vi "Test Namer With Folder Creates Folder.vi"(11 "Test Case In":refnum<class "Namer Tests.lvclass">) -> (0 "error out":errorcluster, 3 "Test Case Out":refnum<class "Namer Tests.lvclass">)   [LabVIEW 2020, in "Namer Tests.lvclass"]
uses:
  Namer Tests.lvclass
  C:/Program Files/National Instruments/LabVIEW 2026/vi.lib/Astemes/LUnit/Test Case.lvclass
  Source/Approval Tests/Namer with Folder/Namer with Folder.lvclass
  Source/Approval Tests/Naming Data/Naming Data.lvclass
  Source/Approval Tests/Naming Data/Naming Data.lvclass/Naming Data.ctl
  <vilib>/Astemes/LUnit/Test Case.lvclass/Test Case.ctl
  01b65d38-618d-4a61-b092-aeaffa944d44.vi
  62f3f5be-2136-4147-be65-cbbff562f146.vi
  Source/Approval Tests/Naming Data/Write Test VI Name.vi
  <vilib>/Astemes/LUnit/Core/LUnit Test Case/Private/Append Pass Result.vi
  <vilib>/Astemes/LUnit/Core/LUnit Test Case/Private/Append Fail Result.vi
  01b65d38-618d-4a61-b092-aeaffa944d44.vi/9c5d11cd-9439-4240-a1ee-d9baace9c924.vi
  62f3f5be-2136-4147-be65-cbbff562f146.vi/9c5d11cd-9439-4240-a1ee-d9baace9c924.vi
  <vilib>/Astemes/LUnit/Core/LUnit Test Case/Private/Run In UI.vi
  <vilib>/Astemes/LUnit/Test Case.lvclass
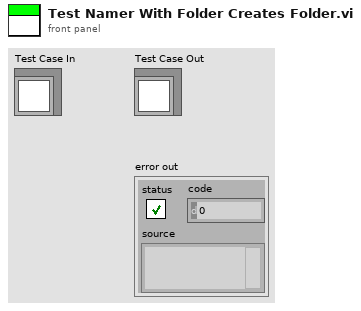
[diagram p1: front panel]
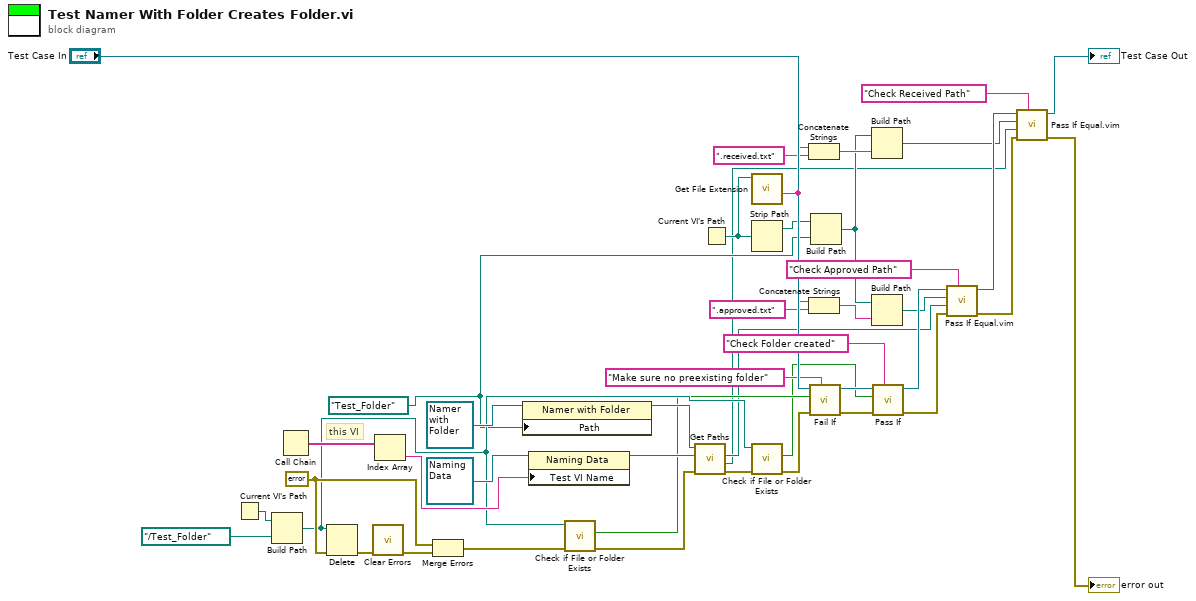
[diagram p0: block diagram]
diagram:
  w14 = path "Test_Folder" ("Path")
  w34 = errorcluster {"status"=FALSE, "code"=0, "source"=""} ("error in (no error)")
  # "this VI"
  n1 = Current VI's Path() -> (path=w35:path)
  n2 = Build Path(base path=w35, name or relative path=path "../Test_Folder") -> (appended path=w28:path)
  n3 = Call Chain() -> (call chain=w40:string[])
  n4 = Delete(path (use dialog)=w28, error in=w34) -> (error out=w33:errorcluster)  [unwired: 3 in, 2 out]
  n5 = call <vilib>:"Clear Errors.vi"("error in (no error)"=w33) -> ("error out"=w32:errorcluster)  [unwired: 5 in, 1 out]
  n6 = Index Array(array=w40) -> (element=w39:string)  [unwired: 1 in]
  n7 = Merge Errors(w34, w32) -> (w30:errorcluster)
  n8 = property class="Namer with Folder"(reference=refnum<class "Namer with Folder.lvclass"> refnum ("Approval Tests:Namer with Folder.lvclass"), "Path"=w14) -> (reference out=w37:refnum<class "Namer with Folder.lvclass">)  [unwired: 1 in, 1 out]
  n9 = property on="Property Node" class="Naming Data"(reference=refnum<class "Naming Data.lvclass"> refnum ("Naming Data"), "Test VI Name"=w39) -> (reference out=w38:refnum<class "Naming Data.lvclass">)  [unwired: 1 in, 1 out]
  n10 = call <vilib>:"Check if File or Folder Exists.vi"("error in (no error)"=w30, "path"=w28) -> ("error out"=w29:errorcluster, "file or folder exists?"=w27:bool)  [unwired: 7 in, 1 out]
  n11 = call-dynamic "Get Paths.vi"("error in"=w29, "Naming Data"=w38, "Namer with Folder in"=w37) -> ("error out"=w31:errorcluster, "Received Path"=w5:path, "Approved Path"=w6:path)  [unwired: 5 in, 1 out]
  n12 = Current VI's Path() -> (path=w22:path)
  n13 = call <vilib>:"Get File Extension.vi"("file"=w22) -> ("filename without extension"=w21:string)  [unwired: 6 in, 4 out]
  n14 = Strip Path(path=w22) -> (stripped path=w15:path)  [unwired: 1 out]
  n15 = call <vilib>:"Check if File or Folder Exists.vi"("error in (no error)"=w31, "path"=w28) -> ("error out"=w13:errorcluster, "file or folder exists?"=w23:bool)  [unwired: 7 in, 1 out]
  n16 = Concatenate Strings(w21, ".received.txt" ("string")) -> (w18:string)
  n17 = Concatenate Strings(w21, ".approved.txt" ("string")) -> (w17:string)
  n18 = call <vilib>:"Fail If.vi"("Description"="Make sure no preexisting folder" ("Label"), "error in (no error)"=w13, "Fail?"=w27, "LUnit Test Case In"="Test Case In") -> ("error out"=w43:errorcluster, "LUnit Test Case Out"=w25:refnum<class "Namer Tests.lvclass">)  [unwired: 6 in]
  n19 = Build Path(base path=w15, name or relative path=w14) -> (appended path=w16:path)
  n20 = Build Path(base path=w16, name or relative path=w18) -> (appended path=w4:path)
  n21 = Build Path(base path=w16, name or relative path=w17) -> (appended path=w3:path)
  n22 = call <vilib>:"Pass If.vi"("Description"="Check Folder created" ("Label (VI Title)"), "error in (no error)"=w43, "Pass?"=w23, "LUnit Test Case In"=w25) -> ("error out"=w8:errorcluster, "LUnit Test Case Out"=w12:refnum<class "Namer Tests.lvclass">)  [unwired: 6 in]
  n23 = call "Pass If Equal.vim"("Description"="Check Approved Path", "error in (no error)"=w8, "Actual"=w6, "Expected"=w3, "LUnit Test Case In"=w12) -> ("error out"=w7:errorcluster, "LUnit Test Case Out"=w10:refnum<class "Namer Tests.lvclass">)  [unwired: 5 in]
  n24 = call "Pass If Equal.vim"("Description"="Check Received Path", "error in (no error)"=w7, "Actual"=w5, "Expected"=w4, "LUnit Test Case In"=w10) -> ("error out"=→"error out":errorcluster, "LUnit Test Case Out"=→"Test Case Out":refnum<class "Namer Tests.lvclass">)  [unwired: 5 in]
